vi "Parse Target for Classes.vi"(7 "exclude dependencies":bool=TRUE, 8 "error in":errorcluster, 11 "target reference":refnum<vi>) -> (0 "error out":errorcluster, 3 "Plant UML String":string)   [LabVIEW 2021, in "TAF Proj Document Type.lvlib" / "Project Parser.lvlib"]
uses:
  <vilib>/Wovalab/AntiDoc/Document Type/Add-ons/LabVIEW TAF Project/Project Parser/Project Parser.lvlib
  <vilib>/Wovalab/AntiDoc/classy-diagram-viewer/classyDiagramViewer.lvlib
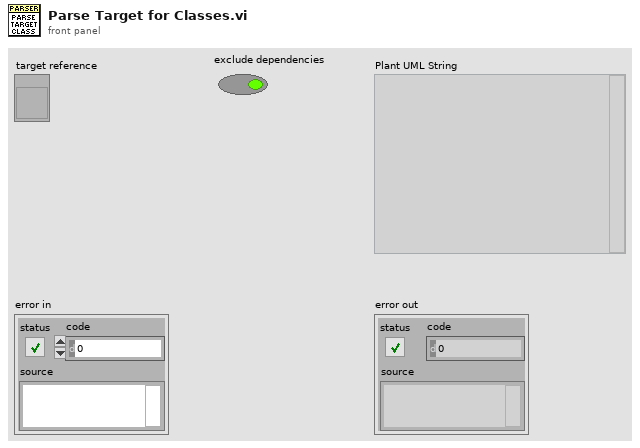
[diagram p1: front panel]
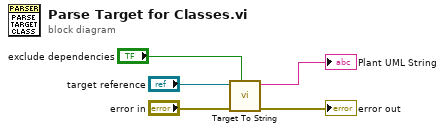
[diagram p0: block diagram]
diagram:
  n1 = call <vilib>:"Target To String.vi"("exclude dependencies"="exclude dependencies", "error in (no error)"="error in", "target reference"="target reference") -> ("error out"=→"error out":errorcluster, "plantUML string"=→"Plant UML String":string)  [unwired: 7 in]
